vi "GUI Set Error To String.vi"(2 "error in (no error)":errorcluster, 3 "label(s) (status)":string="status") -> ()   [LabVIEW 2018]
doc: "Displays error in the string referenced by its label. The string object must be first registered by the SGUI lib."
uses:
  varilib/SGUI Assign Multiple Strings With Tags By Label.vi
  varilib/varilib.lvlib
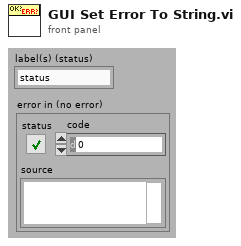
[diagram p1: front panel]
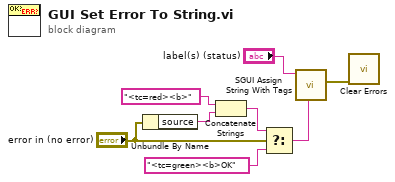
[diagram p0: block diagram]
diagram:
  n1 = Unbundle By Name("error in (no error)") -> ("source"=w1:string)
  n2 = Concatenate Strings("<tc=red><b>" ("string"), w1) -> (w6:string)
  n3 = Select(t=w6, s="error in (no error)", f="<tc=green><b>OK") -> (s? t:f=w4:string)
  n4 = call-poly "SGUI Assign String With Tags.vi"("label(s) (empty)"="label(s) (status)", "string (empty)"=w4) -> ("error out"=w3:errorcluster)  [unwired: 8 in, 1 out]
  n5 = call <vilib>:"Clear Errors.vi"("error in (no error)"=w3) -> ()  [unwired: 5 in, 2 out]
